vi "ge_TableDefaults.vi"(5 "Timing Engine":T2, 7 "ge_TableCmnds":T3, 8 "error in":errorcluster, 9 "ge_DAQManDefinitions":T1, 10 "ChanGrp.lvclass":refnum<class "ChanGrp.lvclass">, 11 "Chan Table":refnum<vi>) -> (0 "error out":errorcluster, 3 "Chan Table Out":refnum<vi>)   [LabVIEW 2018]
uses:
  Classes/Cfg Grandmaster/Class Chan Group/ChanGrp.lvclass
  Custom Ctls Table/ge_TableCmnds.ctl
  Common/Controls/TE_Designator.ctl
  Common/Controls/DAQMan Definitions.ctl
  Classes/Cfg Grandmaster/Class Chan Group/Read MeasType.vi
  Classes/Cfg Grandmaster/Class Chan Group/Read GroupChans.vi
  Classes/Measurements/Class Channel/Read Device.vi
  Classes/Measurements/Class Channel/Channel.lvclass
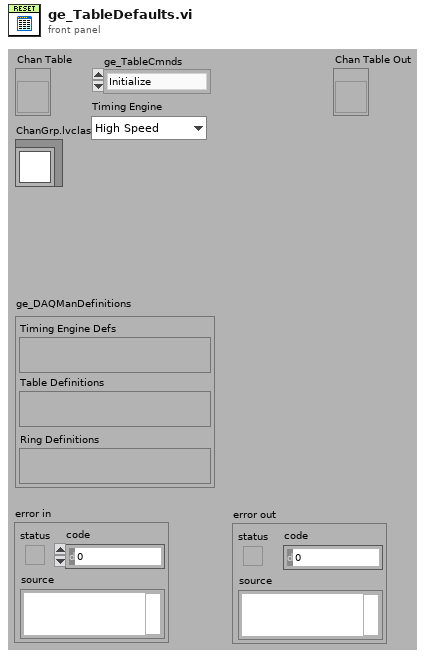
[diagram p1: front panel]
types:
  T1 = typedef "DAQMan Definitions.ctl" = cluster{"Timing Engine Defs":variant, "Table Definitions":variant, "Ring Definitions":variant}
  T2 = typedef "TE_Designator.ctl" = enum16{"High Speed", "Low Speed"}
  T3 = typedef "ge_TableCmnds.ctl" = enum16{"Initialize", "Hide Cell Ctrls", "Position Ctrls", "Load Table", "Reset Table", "Clear Selections", "Ungchd Enter?", "Cell ValChng", "Click Ring", "Edit Cell", "Dismiss Menu", "Glbl Apply", "Calibrate", "Apply Settings", "Cell Key", "SaveChanList", "LoadChanDesc", "Shutdown"}
  T4 = typedef "ge_MeasType.ctl" = enum16{"Voltage", "Frequency", "Tachometer", "Dynamic", "Thermocouple", "RTD", "Strain", "Current", "Resistance"}
  T5 = typedef "ge_ColDef.ctl" = cluster{"ge_HdrNames":T6, "HdrInfo":T7}
  T6 = typedef "HeaderNames.ctl" = enum16{"Channel", "Device", "Spacer", "Description", "MB", "Range", "Terminal", "Coupling", "Thresh (V)", "Pulse/Rev", "Slope", "Min EU", "Min RPM", "mV/EU", "Iex", "Temp Units", "Type", "CJC Src", "CJC Val", "Ro", "Wire Cfg", "Strain Mode", "Vex", "Bridge Type", "GF", "Gauge Res", "Poisson", "Lead Res", "Init Strain", "GAF", "Scale", "Offset", "Unit (EU)", "dB?", "dB Ref", "Cal Mag", "Cal Units", "Max Temp", "Min Temp", "Max Strain", "Min Strain"}
  T7 = typedef "ge_HdrInfo.ctl" = cluster{"Hdr Width":i32, "Glbl Ctrl":T8}
  T8 = typedef "ge_GlblCtrls.ctl" = enum16{"Str0", "Bool0", "Bool1", "Int0", "Ring0", "Ring1", "Ring2", "Ring3", "Dbl0", "Dbl1", "Dbl2", "Dbl3", "Cal0", "Cal1", "Cal2", "None"}
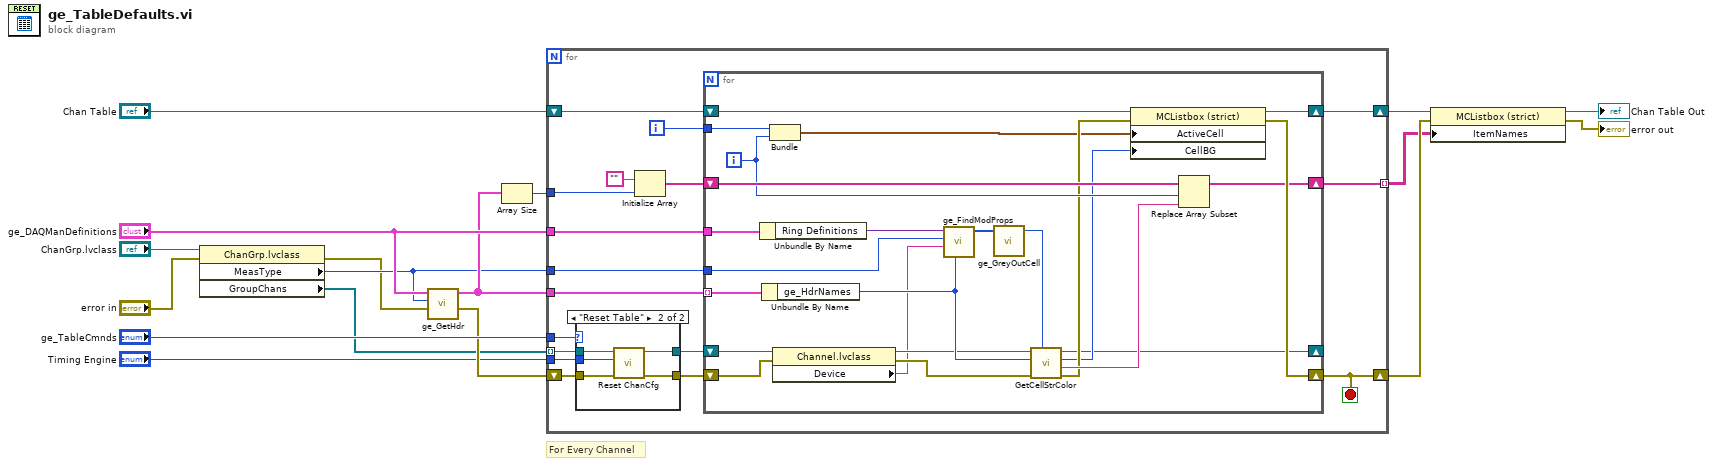
[diagram p0: block diagram]
diagram:
  # "For Every Channel"
  n1 = property class="ChanGrp.lvclass"(reference="ChanGrp.lvclass", error in="error in") -> (error out=w2:errorcluster, "MeasType"=w4:T4, "GroupChans"=w1:refnum<class "Channel.lvclass">[])  [unwired: 1 out]
  n2 = call "ge_GetHdr.vi"("error in"=w2, "MeasType"=w4, "ge_DAQManDefinitions"="ge_DAQManDefinitions") -> ("error out"=w10:errorcluster, "Table Hdrs"=w7:T5[])  [unwired: 7 in]
  n3 = Array Size(array=w7) -> (size(s)=w6:i32)
  n4 = for {
    shift-right: [w32] -> w16
    shift-left: "Chan Table" -> [w33]
    shift-right: [w31] -> w15
    shift-left: w10 -> [w23]
    tunnel: w1 -> [w24] mode=indexing
    tunnel: "ge_TableCmnds" -> [w34]
    tunnel: w7 -> [w29]
    tunnel: [w30] -> w11 mode=indexing
    tunnel: "ge_DAQManDefinitions" -> [w25]
    tunnel: "Timing Engine" -> [w22]
    tunnel: w4 -> [w21]
    tunnel: w6 -> [w18]
    i -> [w27]
    stop <- w31 stop-if-true
    n5 = case shown="\"Reset Table\"" w34 {
      tunnel: [w59 w64] -> w28
      tunnel: w24 -> [w59 w65]
      tunnel: w23 -> [w60 w62]
      tunnel: [w60 w63] -> w26
      tunnel: w22 -> [_ w61]
      frame Default {
      }
      frame "Reset Table" {
        n6 = call "Reset ChanCfg.vi"("error in (no error)"=w62, "Timing Engine"=w61, "Channel in"=w65) -> ("error out"=w63:errorcluster, "Channel out"=w64:refnum<class "Channel.lvclass">)  [unwired: 7 in]
      }
    }
    n7 = Initialize Array("", w18) -> (w19:string[])
    n8 = for {
      shift-right: [w52] -> w32
      shift-left: w33 -> [w53]
      shift-right: [w51] -> w31
      shift-left: w26 -> [w58]
      shift-right: [w49] -> w30
      shift-left: w19 -> [w50]
      tunnel: w29 -> [w56] mode=indexing
      tunnel: w27 -> [w54]
      tunnel: w25 -> [w46]
      tunnel: w21 -> [w45]
      shift-right: [w35] -> _
      shift-left: w28 -> [w57]
      i -> [w48]
      n9 = Unbundle By Name(w46) -> ("Ring Definitions"=w41:variant)
      n10 = Unbundle By Name(w56) -> ("ge_HdrNames"=w55:T6)
      n11 = Bundle(w54, w48) -> (w36:cluster{i32, i32})  [unwired: 1 in]
      n12 = property class="Channel.lvclass"(reference=w57, error in=w58) -> (reference out=w39:refnum<class "Channel.lvclass">, error out=w40:errorcluster, "Device"=w38:string)
      n13 = call "ge_FindModProps.vi"("Hdr Name"=w55, "Device"=w38, "MeasType"=w45, "All Ring Support"=w41) -> ("Values"=w42:u16[])  [unwired: 6 in, 1 out]
      n14 = call "ge_GreyOutCell.vi"("V Ranges"=w42) -> ("Color"=w37:u32)  [unwired: 4 in]
      n15 = call-dynamic "GetCellStrColor.vi"("Color"=w37, "error in (no error)"=w40, "Hdr Name"=w55, "Channel in"=w39) -> ("error out"=w44:errorcluster, "Cell String"=w47:string, "Cell Color"=w43:u32, "Channel out"=w35:refnum<class "Channel.lvclass">)  [unwired: 4 in]
      n16 = property on="Property Node" class="MCListbox (strict)"(reference=w53, error in=w44, "ActiveCell"=w36, "CellBG"=w43) -> (reference out=w52:refnum<vi>, error out=w51:errorcluster)
      n17 = Replace Array Subset(array=w50, new element=w47, index=w48) -> (w49:string[])
    }
  }
  n18 = property on="Property Node" class="MCListbox (strict)"(reference=w16, error in=w15, "ItemNames"=w11) -> (reference out=→"Chan Table Out":refnum<vi>, error out=→"error out":errorcluster)
